vi "Configuration_to_Array.vi"(11 "file (use dialog)":path) -> (2 "Table Control":string[][](table))   [LabVIEW 2020]
uses:
  <vilib>/Utility/file.llb/Read Delimited Spreadsheet (string).vi
panel:
  out "Device Name":string
  out "initialized array":string[](array[string])
  out "Value":string
  out "Attribute":string
  out "element":string
  out "all rows":string[][](array[string])
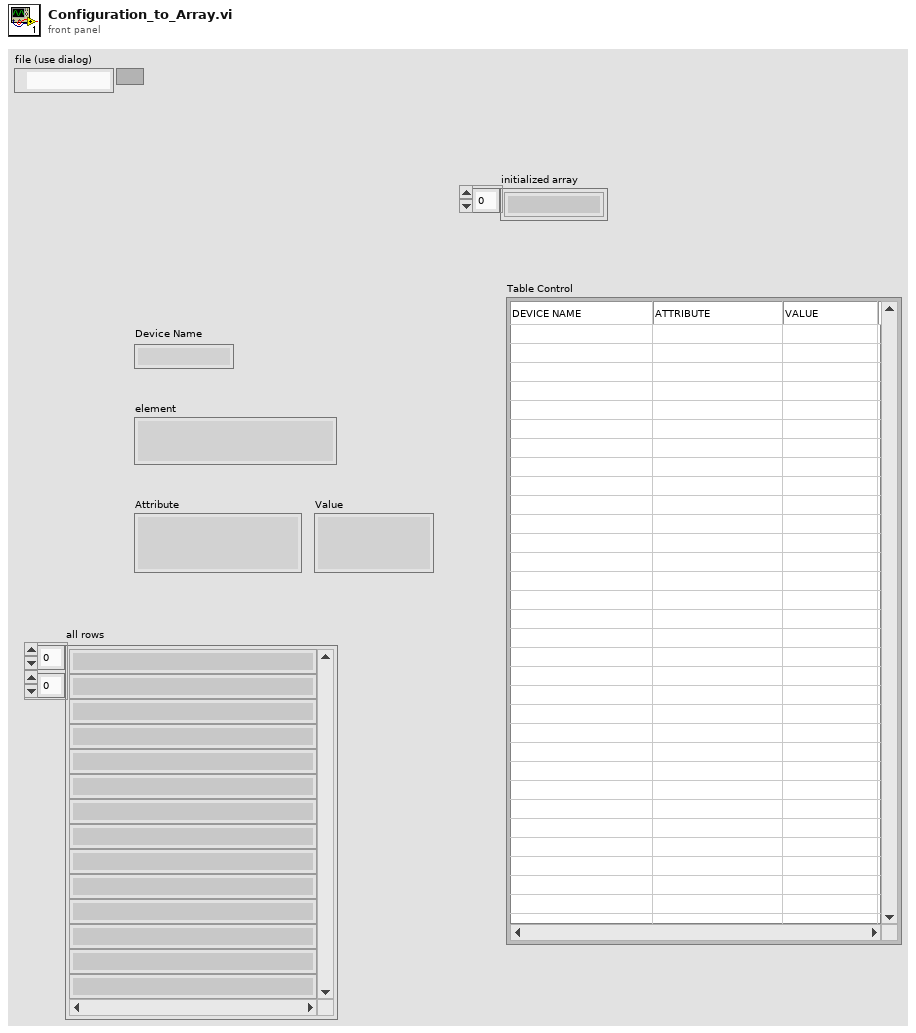
[diagram p1: front panel]
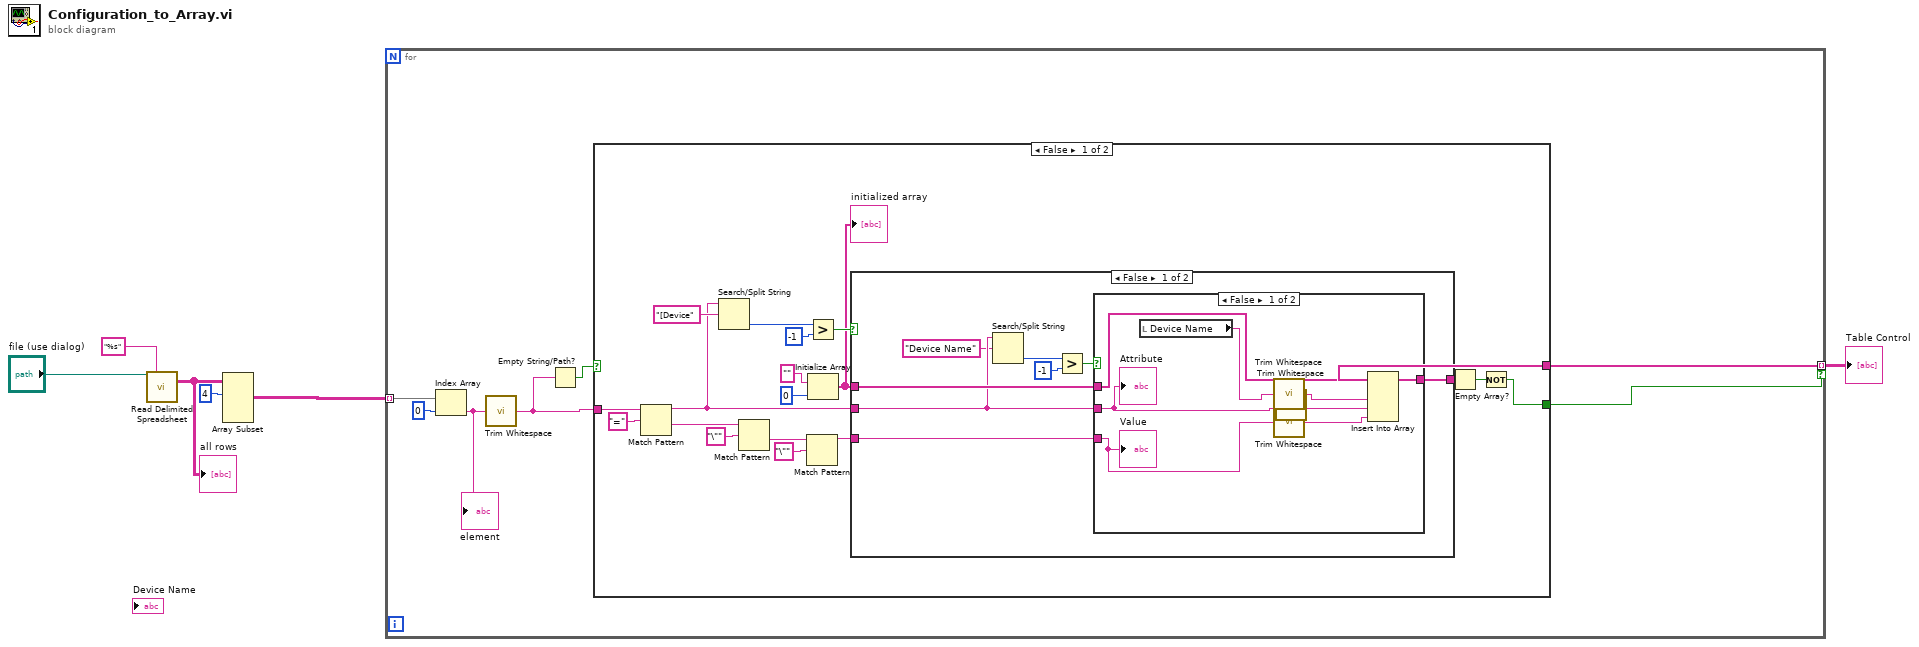
[diagram p0: block diagram]
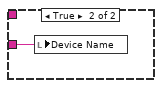
[diagram p2: hidden frame]
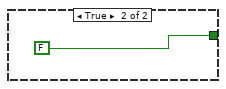
[diagram p4: hidden frame]
diagram:
  n1 = call-poly <vilib>:"Read Delimited Spreadsheet.vi"("file path (dialog if empty)"="file (use dialog)", "format (%s)"="%s") -> ("all rows"=w4:string[][])  [unwired: 8 in, 5 out]
  "all rows" <- w4
  n2 = Array Subset(array=w4, index (row)=4 ("index")) -> (w2:string[][])  [unwired: 3 in]
  n3 = for {
    tunnel: w2 -> [w12] mode=indexing
    tunnel: [w10] -> w1 mode=indexing if=w9
    n4 = Index Array(array=w12, index=0) -> (element=w11:string)
    "element" <- w11
    n5 = call <vilib>:"Trim Whitespace.vi"("string"=w11) -> ("trimmed string"=w7:string)  [unwired: 1 in]
    n6 = Empty String/Path?(string/path=w7) -> (empty?=w8:bool)
    n7 = case shown="False" w8 {
      tunnel: w7 -> [w31 _]
      tunnel: [w16 _] -> w10
      tunnel: [w14 FALSE] -> w9
      frame False {
        n8 = Match Pattern(string=w31, regular expression="=") -> (before substring=w21:string, after substring=w29:string)  [unwired: 1 in, 2 out]
        n9 = Search/Split String(string=w21, search string/char (-)="[Device") -> (offset of match=w24:i32)  [unwired: 1 in, 2 out]
        n10 = Match Pattern(string=w29, regular expression="\"") -> (after substring=w26:string)  [unwired: 1 in, 3 out]
        n11 = Match Pattern(string=w26, regular expression="\"") -> (before substring=w20:string)  [unwired: 1 in, 3 out]
        n12 = Greater?(x=w24, y=-1) -> (0:w22:bool)
        n13 = Initialize Array("" ("regular expression"), 0 ("dimension size")) -> (w18:string[])
        "initialized array" <- w18
        n14 = case shown="False" w22 {
          tunnel: w21 -> [w35 _]
          tunnel: w20 -> [w38 _]
          tunnel: w18 -> [w39 _]
          tunnel: [w32 _] -> w16
          frame False {
            n15 = Search/Split String(string=w35, search string/char (-)="Device Name") -> (offset of match=w37:i32)  [unwired: 1 in, 2 out]
            n16 = Greater?(x=w37, y=-1) -> (0:w33:bool)
            n17 = case shown="False" w33 {
              tunnel: w39 -> [w47 _]
              tunnel: w35 -> [w43 _]
              tunnel: w38 -> [w42 w48]
              tunnel: [w46 _] -> w32
              frame False {
                n18 = local read "Device Name"() -> (w45:string)
                n19 = call <vilib>:"Trim Whitespace.vi"("string"=w45) -> ("trimmed string"=w44:string)  [unwired: 1 in]
                n20 = call <vilib>:"Trim Whitespace.vi"("string"=w42) -> ("trimmed string"=w40:string)  [unwired: 1 in]
                n21 = call <vilib>:"Trim Whitespace.vi"("string"=w43) -> ("trimmed string"=w41:string)  [unwired: 1 in]
                n22 = Insert Into Array(array=w47, new element #1=w44, new element #2=w41, new element #3=w40) -> (w46:string[])  [unwired: 1 in]
                "Attribute" <- w43
                "Value" <- w42
              }
              frame True {
                n23 = local write "Device Name"(w48) -> ()
              }
            }
          }
          frame True {
          }
        }
        n24 = Empty Array?(array=w16) -> (empty?=w15:bool)
        n25 = Not(x=w15) -> (.not. x?=w14:bool)
      }
      frame True {
      }
    }
  }
  "Table Control" <- w1
